vi "ConfigureSequence.vi"(0 "object in":refnum<class "Hamamatsu.lvclass">, 2 "Sequence Settings":T1={"Master Pulse Settings"={"Mode"=1, "Source"=1, "Interval"=1.0, "Burst"=0}, "Capture mode"=0, "Frames"=0, "Dcam Trigger Source"=1, "External Options"={"Polarity"=1, "Delay"=0.0}, "ExposureTime(ms)"=0.0} {"External Options"."Polarity" items=["Negative"=1, "Positive"=2]; "Dcam Trigger Source" items=["Internal"=1, "External"=2, "Software"=3, "Master Pulse"=4]; "Capture mode" items=["Snap", "Sequence"]; "Master Pulse Settings"."Source" items=["External"=1, "Software"=2]; "Master Pulse Settings"."Mode" items=["Continuous"=1, "Start"=2, "Burst"=3]}, 3 "globalshutter":bool, 5 "error in (no error)":errorcluster) -> (14 "object out":refnum<class "Hamamatsu.lvclass">, 19 "error out":errorcluster)   [LabVIEW 2024, in "Hamamatsu.lvclass"]
uses:
  Hamamatsu.lvclass
  Hamamatsu.lvclass/Hamamatsu.ctl
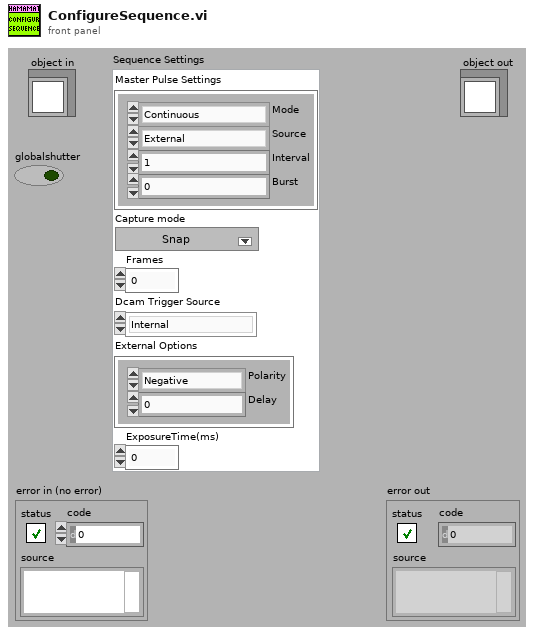
[diagram p1: front panel]
types:
  T1 = cluster{"Master Pulse Settings":cluster{"Mode":u32, "Source":u32, "Interval":dbl, "Burst":u32}, "Capture mode":i32, "Frames":i32, "Dcam Trigger Source":i32, "External Options":cluster{"Polarity":i32, "Delay":dbl}, "ExposureTime(ms)":dbl}
  T2 = cluster{"Mode":u32, "Source":u32, "Interval":dbl, "Burst":u32}
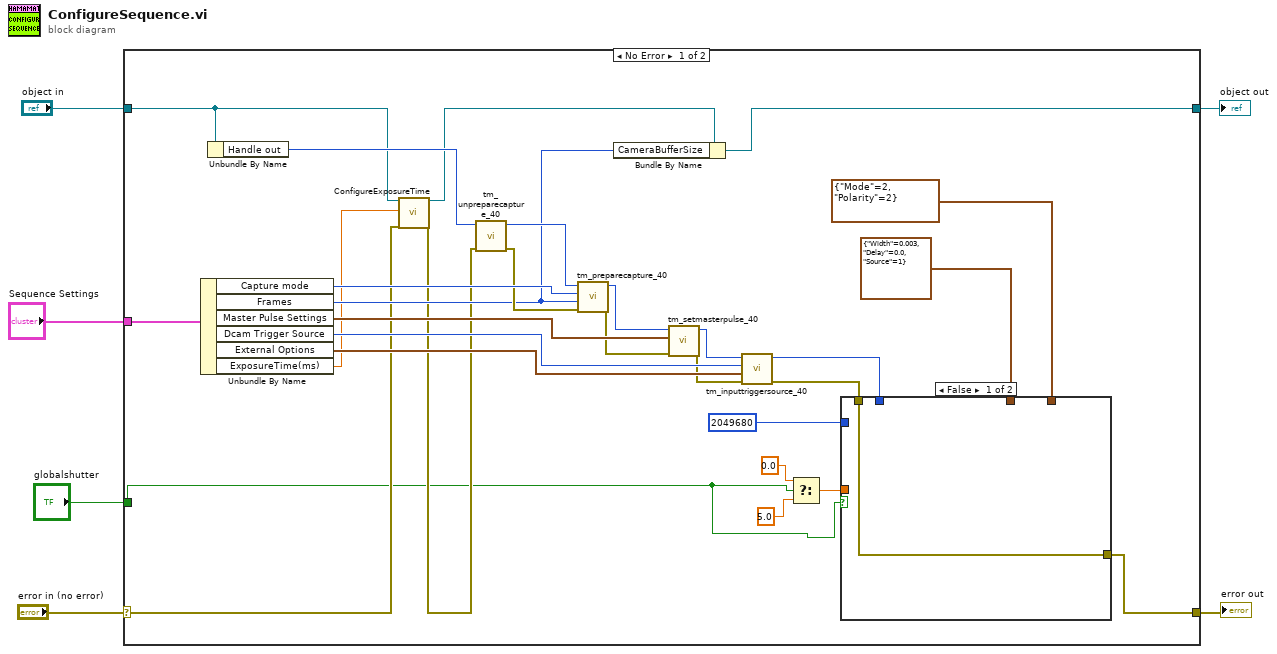
[diagram p0: block diagram]
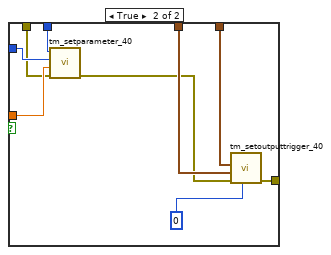
[diagram p2: hidden frame]
diagram:
  n1 = case shown="No Error" "error in (no error)" {
    selector: "error in (no error)" -> [w19 w47]
    tunnel: [w8 w47] -> w5
    tunnel: [w23 w46] -> w3
    tunnel: "object in" -> [w20 w46]
    tunnel: "Sequence Settings" -> [w35 _]
    tunnel: "globalshutter" -> [w7 _]
    frame No Error {
      n2 = Unbundle By Name(w35) -> ("Capture mode"=w34:i32, "Frames"=w22:i32, "Master Pulse Settings"=w32:T2, "Dcam Trigger Source"=w29:i32, "External Options"=w28:cluster{"Polarity":i32, "Delay":dbl}, "ExposureTime(ms)"=w17:dbl)
      n3 = Unbundle By Name(w20) -> ("Handle out"=w26:u32)
      n4 = call-dynamic "ConfigureExposureTime.vi"("object in"=w20, "ExposureTime(ms)"=w17, "error in (no error)"=w19) -> ("object out"=w21:refnum<class "Hamamatsu.lvclass">, "error out"=w18:errorcluster)  [unwired: 15 in]
      n5 = call <userlib>:"tm_unpreparecapture_40.vi"("error in (no error)"=w18, "Handle in"=w26) -> ("error out"=w25:errorcluster, "Handle out"=w24:u32)  [unwired: 8 in]
      n6 = call <userlib>:"tm_preparecapture_40.vi"("error in (no error)"=w25, "Frames"=w22, "Capture mode"=w34, "Handle in"=w24) -> ("error out"=w31:errorcluster, "Handle out"=w33:u32)  [unwired: 4 in, 2 out]
      n7 = Bundle By Name(cluster=w21, "CameraBufferSize"=w22) -> (w23:refnum<class "Hamamatsu.lvclass">)
      n8 = call <userlib>:"tm_setmasterpulse_40.vi"("error in (no error)"=w31, "Parameters"=w32, "Handle in"=w33) -> ("error out"=w27:errorcluster, "Handle out"=w30:u32)  [unwired: 7 in]
      n9 = call <userlib>:"tm_inputtriggersource_40.vi"("error in (no error)"=w27, "External Options"=w28, "Source"=w29, "Handle in"=w30) -> ("error out"=w9:errorcluster, "Handle out"=w15:u32)  [unwired: 6 in]
      n10 = Select(t=0.0, s=w7, f=5.0) -> (s? t:f=w14:dbl)
      n11 = case shown="False" w7 {
        tunnel: 2049680 ("Frames to Capture 2") -> [_ w45]
        tunnel: w15 -> [_ w44]
        tunnel: w14 -> [_ w43]
        tunnel: cluster{"Width":dbl, "Delay":dbl, "Source":u32} {"Width"=0.003, "Delay"=0.0, "Source"=1} ("Programmable Options") -> [_ w41]
        tunnel: cluster{"Mode":u32, "Polarity":u32} {"Mode"=2, "Polarity"=2} ("Type") -> [_ w40]
        tunnel: w9 -> [w36 w39]
        tunnel: [w36 w37] -> w8
        frame False {
        }
        frame True {
          n12 = call <userlib>:"tm_setparameter_40.vi"("error in (no error)"=w39, "Value in"=w43, "Parameter"=w45, "Handle in"=w44) -> ("error out"=w38:errorcluster)  [unwired: 6 in, 1 out]
          n13 = call <userlib>:"tm_setoutputtrigger_40.vi"("Port"=0, "error in (no error)"=w38, "Programmable Options"=w41, "Type"=w40) -> ("error out"=w37:errorcluster)  [unwired: 6 in, 1 out]
        }
      }
    }
    frame Error {
    }
  }
  "error out" <- w5
  "object out" <- w3
